vi "TSM SSC Digital PPMU Measure Current.vi"(0 "Digital TSM In":T1, 11 "error in":errorcluster) -> (4 "Digital TSM out":T1, 6 "Per-Site Per-Pin Measurements (A)":dbl[][](array[numeric]), 15 "error out":errorcluster)   [LabVIEW 2020]
doc: "Instructs the PPMU to measure current on the specified pin(s) and pin group(s) and returns per-site per-pin current measurements."
uses:
  TSM/TSM SSC Digital.ctl
  <vilib>/NI_TestStand_SemiconductorModule/NI_TestStand_Semiconductor_Module.lvlibp/PinMap/Digital Pattern/PinQueryContext/DigitalPatternPinQueryContext.lvclass
  SSC Digital/SSC Digital.ctl
  <instrlib>/niDigital/niDigital.llb/niDigital Measurement Type.ctl
  b581fc96-8b34-480a-99d0-0b5fa856aaa9.vi
  Shared SubVIs/Channel List to Pins.vi
  Shared SubVIs/Trim Whitespace [Inlined].vi
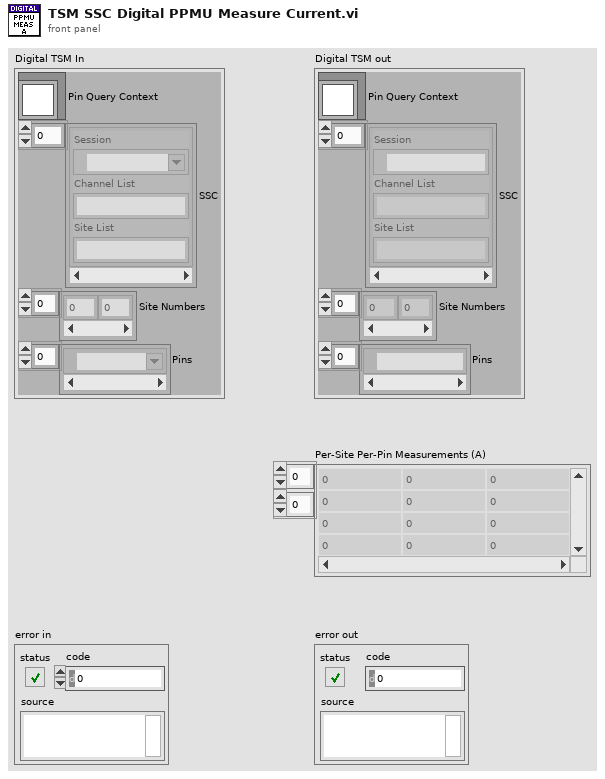
[diagram p1: front panel]
types:
  T1 = typedef "TSM SSC Digital.ctl" = cluster{"Pin Query Context":refnum<class "DigitalPatternPinQueryContext.lvclass">, "SSC":T2[], "Site Numbers":i32[], "Pins":tag[]}
  T2 = typedef "SSC Digital.ctl" = cluster{"Session":refnum<k15>, "Channel List":string, "Site List":string}
  T3 = typedef "niDigital Measurement Type.ctl" = i32
  T4 = typedef "Digital 2D Location Array in a Cluster.ctl" = cluster{"Digital 2D Location Array":T5[]}
  T5 = typedef "Digital 2D Location.ctl" = cluster{"Row":i32, "Col":i32}
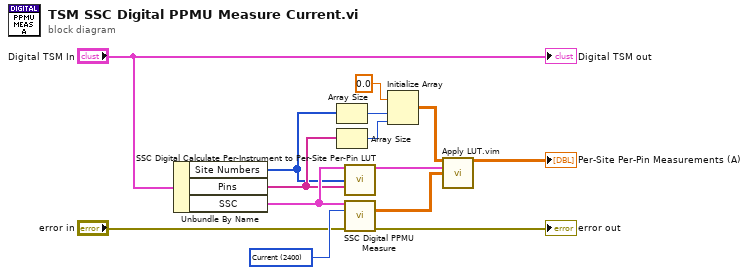
[diagram p0: block diagram]
diagram:
  w5 = T3 2400 items=["Voltage"=2401, "Current"=2400] ("measurement type")
  n1 = Unbundle By Name("Digital TSM In") -> ("Site Numbers"=w9:i32[], "Pins"=w10:tag[], "SSC"=w14:T2[])
  n2 = Array Size(array=w9) -> (size(s)=w6:i32)
  n3 = Array Size(array=w10) -> (size(s)=w7:i32)
  n4 = call "SSC Digital Calculate Per-Instrument to Per-Site Per-Pin LUT.vi"("Digital SSC In"=w14, "Sites"=w9, "Pins"=w10) -> ("Per-Instrument to Per-Site Per-Pin LUT"=w8:T4[])  [unwired: 12 in]
  n5 = call "SSC Digital PPMU Measure.vi"("Digital SSC in"=w14, "Measurement Type"=w5, "error in"="error in") -> ("Per-Instrument Measurements"=w13:dbl[][], "error out"=→"error out":errorcluster)  [unwired: 10 in, 1 out]
  n6 = Initialize Array(0.0 ("element"), w6, w7) -> (w11:dbl[][])
  n7 = call "Apply LUT.vim"("Initialized Array"=w11, "LUT"=w8, "Results to Apply LUT to"=w13) -> ("Array Out"=→"Per-Site Per-Pin Measurements (A)":dbl[][])  [unwired: 12 in]
  "Digital TSM out" <- "Digital TSM In"
